vi "对称性.vi"(11 "XY图":cluster{dbl[], dbl[]}[](graph)) -> (1 "对称性 3":dbl, 2 "对称性 2":dbl, 3 "对称性":dbl)   [LabVIEW 2018]
uses:
  <vilib>/Analysis/NI_AAL_Geometry.lvlib
panel:
  out "右 3":dbl
  out "左 3":dbl
  out "右 2":dbl
  out "左 2":dbl
  out "右":dbl
  out "左":dbl
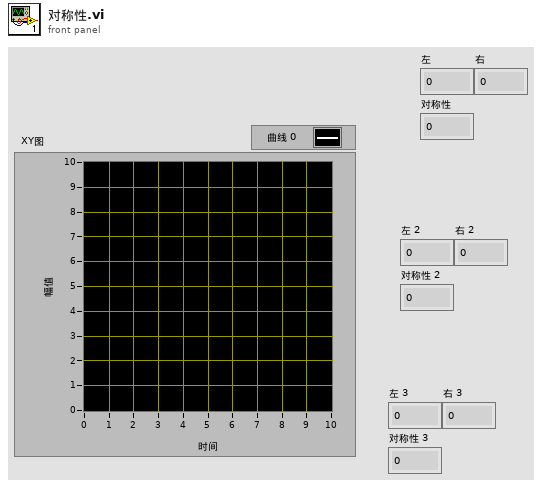
[diagram p1: front panel]
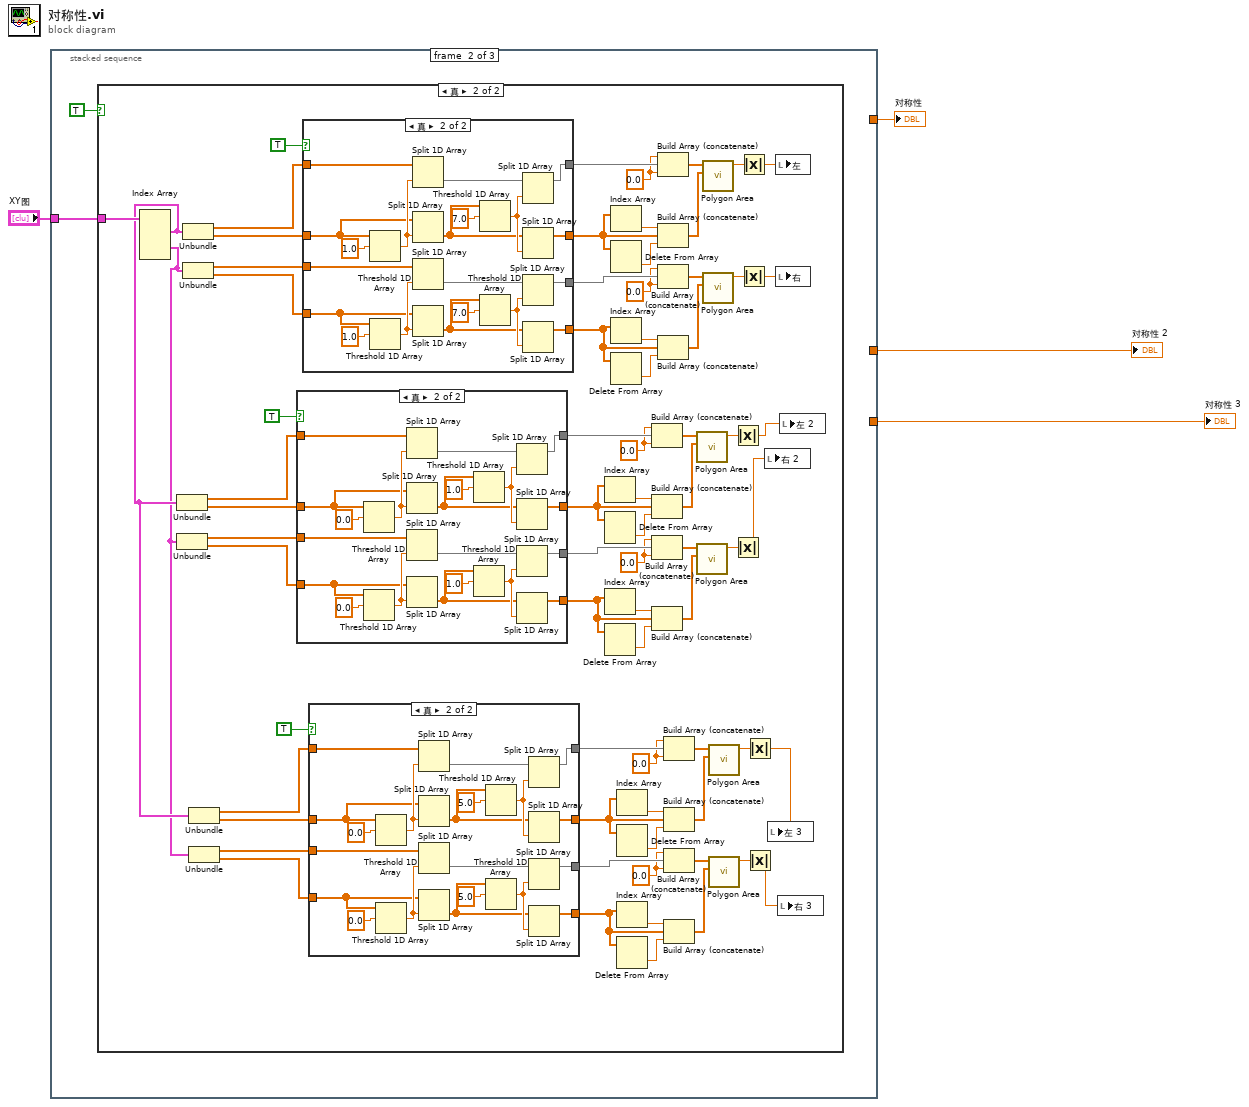
[diagram p0: block diagram]
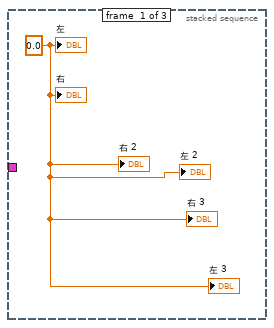
[diagram p2: hidden frame]
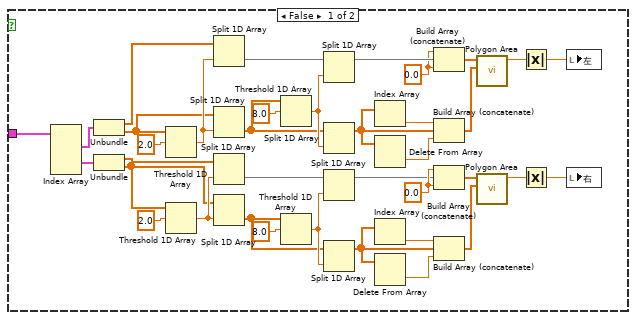
[diagram p3: hidden frame]
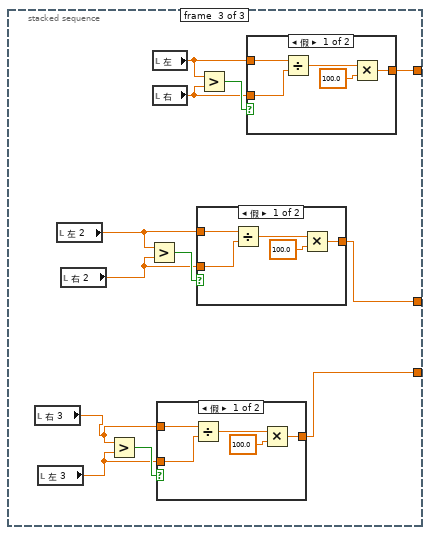
[diagram p7: hidden frame]
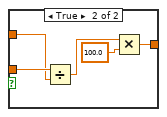
[diagram p8: hidden frame]
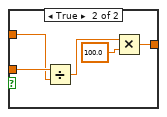
[diagram p9: hidden frame]
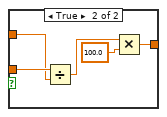
[diagram p10: hidden frame]
diagram:
  n1 = stacked-sequence {
    tunnel: "XY图" -> [_ w6 _]
    tunnel: [_ _ w197] -> w4
    tunnel: [_ _ w190] -> w2
    tunnel: [_ _ w189] -> w1
    frame #0 {
      w5 = 0.0 ("左")
      "左" <- w5
      "右" <- w5
      "右 2" <- w5
      "左 2" <- w5
      "右 3" <- w5
      "左 3" <- w5
    }
    frame #1 {
      n2 = case shown="真" TRUE {
        tunnel: w6 -> [w38 w94]
        frame False {
          w12 = 0.0
          w20 = 0.0
          n3 = Index Array(array=w38) -> (element #1=w39:cluster{dbl[], dbl[]}, element #3=w40:cluster{dbl[], dbl[]})  [unwired: 4 in, 2 out]
          n4 = Unbundle(w39) -> (w36:dbl[], w30:dbl[])
          n5 = Unbundle(w40) -> (w31:dbl[], w32:dbl[])
          n6 = Threshold 1D Array(2:2.0 ("阈值y"), 3:w30) -> (0:w35:dbl)  [unwired: 1 in]
          n7 = Threshold 1D Array(2:2.0 ("阈值y"), 3:w32) -> (0:w34:dbl)  [unwired: 1 in]
          n8 = Split 1D Array(array=w36, index=w35) -> (second subarray=w27:dbl[])  [unwired: 1 out]
          n9 = Split 1D Array(array=w30, index=w35) -> (second subarray=w26:dbl[])  [unwired: 1 out]
          n10 = Split 1D Array(array=w31, index=w34) -> (second subarray=w23:dbl[])  [unwired: 1 out]
          n11 = Split 1D Array(array=w32, index=w34) -> (second subarray=w22:dbl[])  [unwired: 1 out]
          n12 = Threshold 1D Array(2:8.0 ("阈值y"), 3:w26) -> (0:w29:dbl)  [unwired: 1 in]
          n13 = Threshold 1D Array(2:8.0 ("阈值y"), 3:w22) -> (0:w24:dbl)  [unwired: 1 in]
          n14 = Split 1D Array(array=w27, index=w29) -> (first subarray=w21:dbl[])  [unwired: 1 out]
          n15 = Split 1D Array(array=w26, index=w29) -> (first subarray=w18:dbl[])  [unwired: 1 out]
          n16 = Split 1D Array(array=w23, index=w24) -> (first subarray=w10:dbl[])  [unwired: 1 out]
          n17 = Split 1D Array(array=w22, index=w24) -> (first subarray=w11:dbl[])  [unwired: 1 out]
          n18 = Index Array(array=w18) -> (element=w19:dbl)  [unwired: 1 in]
          n19 = Delete From Array(array=w18) -> (deleted portion=w17:dbl)  [unwired: 2 in, 1 out]
          n20 = Index Array(array=w11) -> (element=w13:dbl)  [unwired: 1 in]
          n21 = Delete From Array(array=w11) -> (deleted portion=w14:dbl)  [unwired: 2 in, 1 out]
          n22 = Build Array (concatenate)(w20, w21, w20) -> (w16:dbl[])
          n23 = Build Array (concatenate)(w19, w18, w17) -> (w15:dbl[])
          n24 = Build Array (concatenate)(w12, w10, w12) -> (w9:dbl[])
          n25 = Build Array (concatenate)(w13, w11, w14) -> (w8:dbl[])
          n26 = call <vilib>:"Polygon Area.vi"("Y"=w15, "X"=w16) -> ("signed area"=w41:dbl)  [unwired: 8 in, 1 out]
          n27 = call <vilib>:"Polygon Area.vi"("Y"=w8, "X"=w9) -> ("signed area"=w43:dbl)  [unwired: 8 in, 1 out]
          n28 = Absolute Value(x=w41) -> (abs(x)=w42:dbl)
          n29 = Absolute Value(x=w43) -> (abs(x)=w44:dbl)
          n30 = local write "左"(w42) -> ()
          n31 = local write "右"(w44) -> ()
        }
        frame True {
          w51 = 0.0
          w50 = 0.0
          w74 = 0.0
          w73 = 0.0
          w96 = 0.0
          w95 = 0.0
          n32 = Index Array(array=w94) -> (element #1=w48:cluster{dbl[], dbl[]}, element #3=w47:cluster{dbl[], dbl[]})  [unwired: 4 in, 2 out]
          n33 = Unbundle(w48) -> (w90:dbl[], w87:dbl[])
          n34 = Unbundle(w47) -> (w88:dbl[], w89:dbl[])
          n35 = Unbundle(w48) -> (w112:dbl[], w109:dbl[])
          n36 = Unbundle(w47) -> (w110:dbl[], w111:dbl[])
          n37 = Unbundle(w48) -> (w67:dbl[], w64:dbl[])
          n38 = Unbundle(w47) -> (w65:dbl[], w66:dbl[])
          n39 = case shown="真" TRUE {
            tunnel: w90 -> [w144 w164]
            tunnel: w89 -> [w141 w161]
            tunnel: w88 -> [w142 w160]
            tunnel: w87 -> [w143 w159]
            tunnel: [w144 w152] -> w86
            tunnel: [w143 w151] -> w84
            tunnel: [w141 w150] -> w78
            tunnel: [w142 w149] -> w77
            frame False {
            }
            frame True {
              n40 = Threshold 1D Array(2:0.0 ("阈值y"), 3:w159) -> (0:w163:dbl)  [unwired: 1 in]
              n41 = Threshold 1D Array(2:0.0 ("阈值y"), 3:w161) -> (0:w162:dbl)  [unwired: 1 in]
              n42 = Split 1D Array(array=w164, index=w163) -> (second subarray=w157:dbl[])  [unwired: 1 out]
              n43 = Split 1D Array(array=w159, index=w163) -> (second subarray=w156:dbl[])  [unwired: 1 out]
              n44 = Split 1D Array(array=w160, index=w162) -> (second subarray=w154:dbl[])  [unwired: 1 out]
              n45 = Split 1D Array(array=w161, index=w162) -> (second subarray=w153:dbl[])  [unwired: 1 out]
              n46 = Threshold 1D Array(2:1.0 ("阈值y"), 3:w156) -> (0:w158:dbl)  [unwired: 1 in]
              n47 = Threshold 1D Array(2:1.0 ("阈值y"), 3:w153) -> (0:w155:dbl)  [unwired: 1 in]
              n48 = Split 1D Array(array=w157, index=w158) -> (first subarray=w152:dbl[])  [unwired: 1 out]
              n49 = Split 1D Array(array=w156, index=w158) -> (first subarray=w151:dbl[])  [unwired: 1 out]
              n50 = Split 1D Array(array=w154, index=w155) -> (first subarray=w149:dbl[])  [unwired: 1 out]
              n51 = Split 1D Array(array=w153, index=w155) -> (first subarray=w150:dbl[])  [unwired: 1 out]
            }
          }
          n52 = case shown="真" TRUE {
            tunnel: w112 -> [w168 w188]
            tunnel: w111 -> [w165 w185]
            tunnel: w110 -> [w166 w184]
            tunnel: w109 -> [w167 w183]
            tunnel: [w168 w176] -> w108
            tunnel: [w167 w175] -> w106
            tunnel: [w165 w174] -> w100
            tunnel: [w166 w173] -> w99
            frame False {
            }
            frame True {
              n53 = Threshold 1D Array(2:1.0 ("阈值y"), 3:w183) -> (0:w187:dbl)  [unwired: 1 in]
              n54 = Threshold 1D Array(2:1.0 ("阈值y"), 3:w185) -> (0:w186:dbl)  [unwired: 1 in]
              n55 = Split 1D Array(array=w188, index=w187) -> (second subarray=w181:dbl[])  [unwired: 1 out]
              n56 = Split 1D Array(array=w183, index=w187) -> (second subarray=w180:dbl[])  [unwired: 1 out]
              n57 = Split 1D Array(array=w184, index=w186) -> (second subarray=w178:dbl[])  [unwired: 1 out]
              n58 = Split 1D Array(array=w185, index=w186) -> (second subarray=w177:dbl[])  [unwired: 1 out]
              n59 = Threshold 1D Array(2:7.0 ("阈值y"), 3:w180) -> (0:w182:dbl)  [unwired: 1 in]
              n60 = Threshold 1D Array(2:7.0 ("阈值y"), 3:w177) -> (0:w179:dbl)  [unwired: 1 in]
              n61 = Split 1D Array(array=w181, index=w182) -> (first subarray=w176:dbl[])  [unwired: 1 out]
              n62 = Split 1D Array(array=w180, index=w182) -> (first subarray=w175:dbl[])  [unwired: 1 out]
              n63 = Split 1D Array(array=w178, index=w179) -> (first subarray=w173:dbl[])  [unwired: 1 out]
              n64 = Split 1D Array(array=w177, index=w179) -> (first subarray=w174:dbl[])  [unwired: 1 out]
            }
          }
          n65 = case shown="真" TRUE {
            tunnel: w67 -> [w120 w140]
            tunnel: w66 -> [w117 w137]
            tunnel: w65 -> [w118 w136]
            tunnel: w64 -> [w119 w135]
            tunnel: [w120 w128] -> w63
            tunnel: [w119 w127] -> w61
            tunnel: [w117 w126] -> w55
            tunnel: [w118 w125] -> w54
            frame False {
            }
            frame True {
              n66 = Threshold 1D Array(2:0.0 ("阈值y"), 3:w135) -> (0:w139:dbl)  [unwired: 1 in]
              n67 = Threshold 1D Array(2:0.0 ("阈值y"), 3:w137) -> (0:w138:dbl)  [unwired: 1 in]
              n68 = Split 1D Array(array=w140, index=w139) -> (second subarray=w133:dbl[])  [unwired: 1 out]
              n69 = Split 1D Array(array=w135, index=w139) -> (second subarray=w132:dbl[])  [unwired: 1 out]
              n70 = Split 1D Array(array=w136, index=w138) -> (second subarray=w130:dbl[])  [unwired: 1 out]
              n71 = Split 1D Array(array=w137, index=w138) -> (second subarray=w129:dbl[])  [unwired: 1 out]
              n72 = Threshold 1D Array(2:5.0 ("阈值y"), 3:w132) -> (0:w134:dbl)  [unwired: 1 in]
              n73 = Threshold 1D Array(2:5.0 ("阈值y"), 3:w129) -> (0:w131:dbl)  [unwired: 1 in]
              n74 = Split 1D Array(array=w133, index=w134) -> (first subarray=w128:dbl[])  [unwired: 1 out]
              n75 = Split 1D Array(array=w132, index=w134) -> (first subarray=w127:dbl[])  [unwired: 1 out]
              n76 = Split 1D Array(array=w130, index=w131) -> (first subarray=w125:dbl[])  [unwired: 1 out]
              n77 = Split 1D Array(array=w129, index=w131) -> (first subarray=w126:dbl[])  [unwired: 1 out]
            }
          }
          n78 = Index Array(array=w84) -> (element=w85:dbl)  [unwired: 1 in]
          n79 = Delete From Array(array=w84) -> (deleted portion=w83:dbl)  [unwired: 2 in, 1 out]
          n80 = Index Array(array=w78) -> (element=w79:dbl)  [unwired: 1 in]
          n81 = Delete From Array(array=w78) -> (deleted portion=w80:dbl)  [unwired: 2 in, 1 out]
          n82 = Index Array(array=w106) -> (element=w107:dbl)  [unwired: 1 in]
          n83 = Delete From Array(array=w106) -> (deleted portion=w105:dbl)  [unwired: 2 in, 1 out]
          n84 = Index Array(array=w100) -> (element=w101:dbl)  [unwired: 1 in]
          n85 = Delete From Array(array=w100) -> (deleted portion=w102:dbl)  [unwired: 2 in, 1 out]
          n86 = Index Array(array=w61) -> (element=w62:dbl)  [unwired: 1 in]
          n87 = Delete From Array(array=w61) -> (deleted portion=w60:dbl)  [unwired: 2 in, 1 out]
          n88 = Index Array(array=w55) -> (element=w56:dbl)  [unwired: 1 in]
          n89 = Delete From Array(array=w55) -> (deleted portion=w57:dbl)  [unwired: 2 in, 1 out]
          n90 = Build Array (concatenate)(w73, w86, w73) -> (w82:dbl[])
          n91 = Build Array (concatenate)(w85, w84, w83) -> (w81:dbl[])
          n92 = Build Array (concatenate)(w74, w77, w74) -> (w76:dbl[])
          n93 = Build Array (concatenate)(w79, w78, w80) -> (w75:dbl[])
          n94 = Build Array (concatenate)(w95, w108, w95) -> (w104:dbl[])
          n95 = Build Array (concatenate)(w107, w106, w105) -> (w103:dbl[])
          n96 = Build Array (concatenate)(w96, w99, w96) -> (w98:dbl[])
          n97 = Build Array (concatenate)(w101, w100, w102) -> (w97:dbl[])
          n98 = Build Array (concatenate)(w50, w63, w50) -> (w59:dbl[])
          n99 = Build Array (concatenate)(w62, w61, w60) -> (w58:dbl[])
          n100 = Build Array (concatenate)(w51, w54, w51) -> (w53:dbl[])
          n101 = Build Array (concatenate)(w56, w55, w57) -> (w52:dbl[])
          n102 = call <vilib>:"Polygon Area.vi"("Y"=w81, "X"=w82) -> ("signed area"=w91:dbl)  [unwired: 8 in, 1 out]
          n103 = call <vilib>:"Polygon Area.vi"("Y"=w75, "X"=w76) -> ("signed area"=w92:dbl)  [unwired: 8 in, 1 out]
          n104 = call <vilib>:"Polygon Area.vi"("Y"=w103, "X"=w104) -> ("signed area"=w113:dbl)  [unwired: 8 in, 1 out]
          n105 = call <vilib>:"Polygon Area.vi"("Y"=w97, "X"=w98) -> ("signed area"=w115:dbl)  [unwired: 8 in, 1 out]
          n106 = call <vilib>:"Polygon Area.vi"("Y"=w58, "X"=w59) -> ("signed area"=w68:dbl)  [unwired: 8 in, 1 out]
          n107 = call <vilib>:"Polygon Area.vi"("Y"=w52, "X"=w53) -> ("signed area"=w69:dbl)  [unwired: 8 in, 1 out]
          n108 = Absolute Value(x=w91) -> (abs(x)=w71:dbl)
          n109 = Absolute Value(x=w92) -> (abs(x)=w70:dbl)
          n110 = Absolute Value(x=w113) -> (abs(x)=w114:dbl)
          n111 = Absolute Value(x=w115) -> (abs(x)=w116:dbl)
          n112 = Absolute Value(x=w68) -> (abs(x)=w46:dbl)
          n113 = Absolute Value(x=w69) -> (abs(x)=w45:dbl)
          n114 = local write "右 2"(w70) -> ()
          n115 = local write "左 3"(w46) -> ()
          n116 = local write "左"(w114) -> ()
          n117 = local write "右"(w116) -> ()
          n118 = local write "右 3"(w45) -> ()
          n119 = local write "左 2"(w71) -> ()
        }
      }
    }
    frame #2 {
      n120 = local read "右 3"() -> (w192:dbl)
      n121 = local read "左 3"() -> (w191:dbl)
      n122 = local read "左 2"() -> (w194:dbl)
      n123 = local read "右 2"() -> (w193:dbl)
      n124 = Greater?(x=w192, y=w191) -> (0:w195:bool)
      n125 = Greater?(x=w194, y=w193) -> (0:w196:bool)
      n126 = local read "左"() -> (w198:dbl)
      n127 = local read "右"() -> (w199:dbl)
      n128 = case shown="假" w195 {
        tunnel: w191 -> [w204 w210]
        tunnel: w192 -> [w205 w209]
        tunnel: [w201 w207] -> w189
        frame False {
          n129 = Divide(x=w205, y=w204) -> (x/y=w203:dbl)
          n130 = Multiply(x=w203, y=100.0) -> (x*y=w201:dbl)
        }
        frame True {
          n131 = Divide(x=w210, y=w209) -> (x/y=w208:dbl)
          n132 = Multiply(x=w208, y=100.0) -> (x*y=w207:dbl)
        }
      }
      n133 = case shown="假" w196 {
        tunnel: w193 -> [w214 w220]
        tunnel: w194 -> [w215 w219]
        tunnel: [w211 w217] -> w190
        frame False {
          n134 = Divide(x=w215, y=w214) -> (x/y=w213:dbl)
          n135 = Multiply(x=w213, y=100.0) -> (x*y=w211:dbl)
        }
        frame True {
          n136 = Divide(x=w220, y=w219) -> (x/y=w218:dbl)
          n137 = Multiply(x=w218, y=100.0) -> (x*y=w217:dbl)
        }
      }
      n138 = Greater?(x=w198, y=w199) -> (0:w200:bool)
      n139 = case shown="假" w200 {
        tunnel: w199 -> [w224 w230]
        tunnel: w198 -> [w225 w229]
        tunnel: [w221 w227] -> w197
        frame False {
          n140 = Divide(x=w225, y=w224) -> (x/y=w223:dbl)
          n141 = Multiply(x=w223, y=100.0) -> (x*y=w221:dbl)
        }
        frame True {
          n142 = Divide(x=w230, y=w229) -> (x/y=w228:dbl)
          n143 = Multiply(x=w228, y=100.0) -> (x*y=w227:dbl)
        }
      }
    }
  }
  "对称性" <- w4
  "对称性 2" <- w2
  "对称性 3" <- w1
